vi "Common-ArrayRandomPick.vi"(11 "数组":dbl[](array[numeric])) -> (3 "元素":dbl)   [LabVIEW 2014]
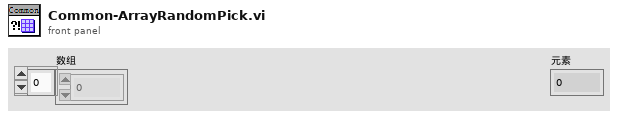
[diagram p1: front panel]
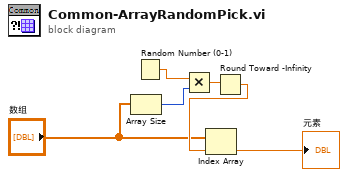
[diagram p0: block diagram]
diagram:
  n1 = Array Size(array="数组") -> (size(s)=w5:i32)
  n2 = Random Number (0-1)() -> (number: 0 to 1=w6:dbl)
  n3 = Multiply(x=w6, y=w5) -> (x*y=w4:dbl)
  n4 = Round Toward -Infinity(1:w4) -> (0:w3:dbl)
  n5 = Index Array(array="数组", index=w3) -> (element=→"元素":dbl)
